vi "moc_en_sygn_SubVi.vi"(11 "signal in":waveform(dbl)) -> (2 "energia":dbl, 3 "Moc sygn okr":dbl)   [LabVIEW 2025]
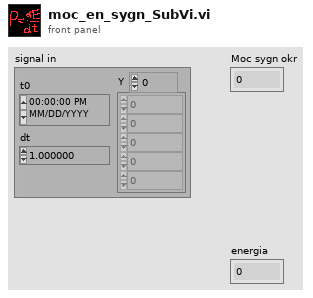
[diagram p1: front panel]
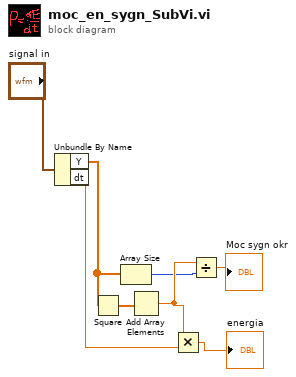
[diagram p0: block diagram]
diagram:
  n1 = Unbundle By Name("signal in") -> ("Y"=w5:dbl[], "dt"=w3:dbl)
  n2 = Square(x=w5) -> (x^2=w2:dbl[])
  n3 = Array Size(array=w5) -> (size(s)=w6:i32)
  n4 = Add Array Elements(numeric array=w2) -> (sum=w7:dbl)
  n5 = Multiply(x=w7, y=w3) -> (x*y=→"energia":dbl)
  n6 = Divide(x=w7, y=w6) -> (x/y=→"Moc sygn okr":dbl)
